vi "ProcessEarlyGvals_1.vi"(0 "G2 vals in":dbl[](array[numeric]) format="%.2f") -> (1 "G2 vals out":dbl[](array[numeric]) format="%.2f", 2 "Tau Values":dbl[](array[numeric])=[0.05, 0.1, 0.15, 0.2, 0.25, 0.3, 0.35, 0.4, 0.45, 0.6, 0.8, 1.0, 1.2, 1.4, 1.6] format="%.2f")   [LabVIEW 2009]
uses:
  <vilib>/Analysis/NI_AALBase.lvlib
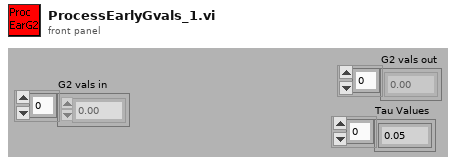
[diagram p1: front panel]
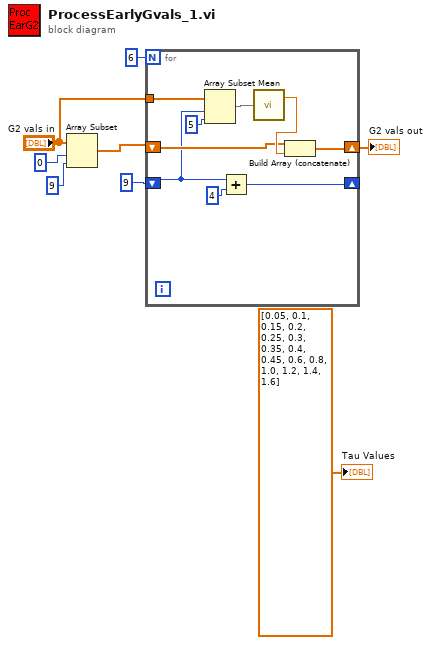
[diagram p0: block diagram]
diagram:
  n1 = Array Subset(array="G2 vals in", index=0, length=9) -> (w6:dbl[])
  n2 = for {
    N: 6 -> [_]
    shift-right: [w12] -> w1
    shift-left: w6 -> [w13]
    tunnel: "G2 vals in" -> [w17]
    shift-right: [w9] -> _
    shift-left: 9 -> [w11]
    n3 = Array Subset(array=w17, index=w11, length=5) -> (w15:dbl[])
    n4 = Add(x=w11, y=4) -> (x+y=w9:i32)
    n5 = call <vilib>:"Mean.vi"("X"=w15) -> ("mean"=w14:dbl)  [unwired: 1 out]
    n6 = Build Array (concatenate)(w13, w14) -> (w12:dbl[])
  }
  "G2 vals out" <- w1
  "Tau Values" <- dbl[] [0.05, 0.1, 0.15, 0.2, 0.25, 0.3, 0.35, 0.4, 0.45, 0.6, 0.8, 1.0, 1.2, 1.4, 1.6]
